vi "Aotunomous constants.vi"() -> (4 "Throttle":dbl, 6 "Wanted Angle":dbl, 8 "Time Of Trigger (S)":dbl, 10 "Time Of Conveyer Belt (S)":dbl, 15 "Power Of Conveyer Belt":dbl)   [LabVIEW 2012]
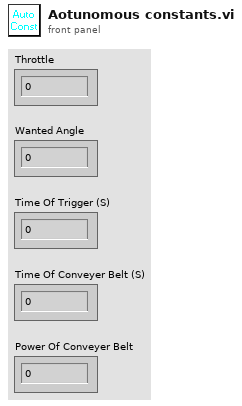
[diagram p1: front panel]
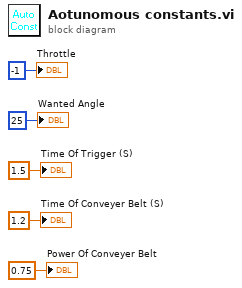
[diagram p0: block diagram]
diagram:
  "Throttle" <- -1
  "Wanted Angle" <- 25
  "Time Of Trigger (S)" <- 1.5
  "Time Of Conveyer Belt (S)" <- 1.2
  "Power Of Conveyer Belt" <- 0.75
